vi "clusters.vi"() -> ()   [LabVIEW 2011]
panel:
  out "Boolean":bool
  out "Numeric 2":dbl
  out "Numeric":dbl
  in  "Cluster":T1
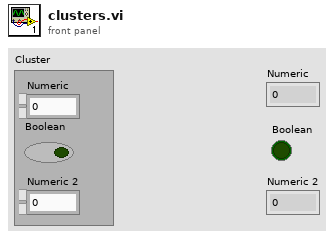
[diagram p1: front panel]
types:
  T1 = cluster{"Numeric":dbl, "Boolean":bool, "Numeric 2":dbl}
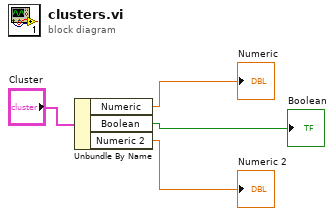
[diagram p0: block diagram]
diagram:
  n1 = Unbundle By Name("Cluster") -> ("Numeric"=→"Numeric":dbl, "Boolean"=→"Boolean":bool, "Numeric 2"=→"Numeric 2":dbl)
